vi "PWVisibleCntl.vi"(5 "Tech":bool, 7 "Product":bool) -> ()   [LabVIEW 2017]
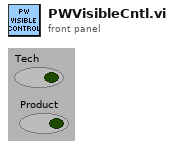
[diagram p1: front panel]
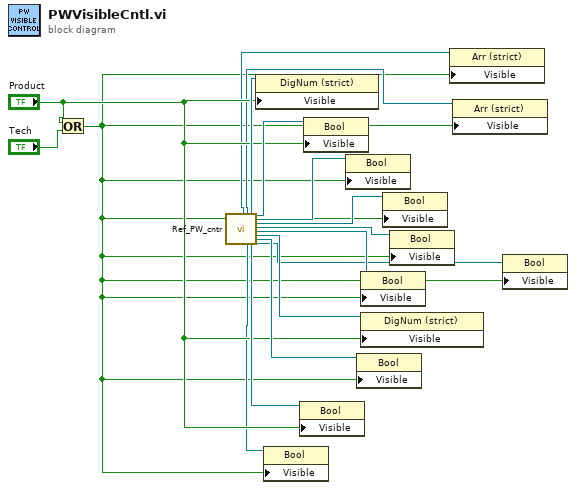
[diagram p0: block diagram]
diagram:
  n1 = Or(x="Product", y="Tech") -> (x .or. y?=w1:bool)
  n2 = call "Ref_PW_cntr.vi"() -> ("Tech.Data Ch out"=w2:refnum<vi>, "Sys Tech.Data S out"=w3:refnum<vi>, "Clear Log out"=w5:refnum<vi>, "I Max Threshold out"=w16:refnum<vi>, "SetOffsetParam out"=w8:refnum<vi>, 20:"Set SN out"=w15:refnum<vi>, "save flash out"=w14:refnum<vi>, "Set Channel Params out"=w13:refnum<vi>, "Set System Params out"=w12:refnum<vi>, "Config. mode out"=w11:refnum<vi>, "I Max OFF Time out"=w10:refnum<vi>, "BackToBootloader out"=w9:refnum<vi>, 27:"Set SN out"=w4:refnum<vi>)  [unwired: 15 in]
  n3 = property class="DigNum (strict)"(reference=w16, "Visible"="Product") -> ()  [unwired: 1 in, 2 out]
  n4 = property class="Bool"(reference=w5, "Visible"=w1) -> ()  [unwired: 1 in, 2 out]
  n5 = property class="Bool"(reference=w8, "Visible"="Product") -> ()  [unwired: 1 in, 2 out]
  n6 = property class="Bool"(reference=w15, "Visible"="Product") -> ()  [unwired: 1 in, 2 out]
  n7 = property class="Bool"(reference=w14, "Visible"=w1) -> ()  [unwired: 1 in, 2 out]
  n8 = property class="Bool"(reference=w9, "Visible"=w1) -> ()  [unwired: 1 in, 2 out]
  n9 = property class="Bool"(reference=w11, "Visible"=w1) -> ()  [unwired: 1 in, 2 out]
  n10 = property class="DigNum (strict)"(reference=w10, "Visible"="Product") -> ()  [unwired: 1 in, 2 out]
  n11 = property class="Bool"(reference=w13, "Visible"=w1) -> ()  [unwired: 1 in, 2 out]
  n12 = property class="Bool"(reference=w12, "Visible"=w1) -> ()  [unwired: 1 in, 2 out]
  n13 = property class="Arr (strict)"(reference=w2, "Visible"=w1) -> ()  [unwired: 1 in, 2 out]
  n14 = property class="Arr (strict)"(reference=w3, "Visible"=w1) -> ()  [unwired: 1 in, 2 out]
  n15 = property class="Bool"(reference=w4, "Visible"=w1) -> ()  [unwired: 1 in, 2 out]
